vi "Tab.Select Page by Name.vi"(8 "Tab Name":string="Page 2", 11 "Tab Control":refnum<vi>) -> ()   [LabVIEW 2018]
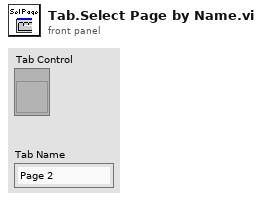
[diagram p1: front panel]
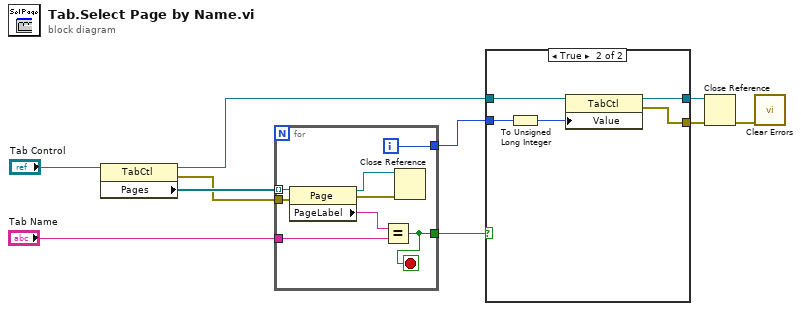
[diagram p0: block diagram]
diagram:
  n1 = property on="Property Node" class="TabCtl"(reference="Tab Control") -> (reference out=w8:refnum<vi>, error out=w9:errorcluster, "Pages"=w10:refnum<vi>[])  [unwired: 1 in]
  n2 = for {
    tunnel: w10 -> [w18] mode=indexing
    tunnel: w9 -> [w15]
    tunnel: [w14] -> w3
    tunnel: "Tab Name" -> [w12]
    tunnel: [w11] -> w2
    i -> [w14]
    stop <- w11 stop-if-true
    n3 = property class="Page"(reference=w18, error in=w15) -> (reference out=w17:refnum<vi>, error out=w16:errorcluster, "PageLabel"=w13:string)
    n4 = Equal?(x=w13, y=w12) -> (x = y?=w11:bool)
    n5 = Close Reference(reference=w17, error in (no error)=w16) -> ()  [unwired: 1 out]
  }
  n6 = case shown="True" w2 {
    tunnel: w8 -> [w19 w24]
    tunnel: [w19 w23] -> w6
    tunnel: [_ w22] -> w5
    tunnel: w3 -> [_ w20]
    frame False {
    }
    frame True {
      n7 = To Unsigned Long Integer(number=w20) -> (unsigned 32bit integer=w21:u32)
      n8 = property on="Property Node" class="TabCtl"(reference=w24, "Value"=w21) -> (reference out=w23:refnum<vi>, error out=w22:errorcluster)  [unwired: 1 in]
    }
  }
  n9 = Close Reference(reference=w6, error in (no error)=w5) -> (error out=w4:errorcluster)
  n10 = call <vilib>:"Clear Errors.vi"("error in (no error)"=w4) -> ()  [unwired: 5 in, 2 out]
